vi "Karma License Activator.vi"() -> ()   [LabVIEW 2022 SP3]
panel:
  in  "Activate License":bool
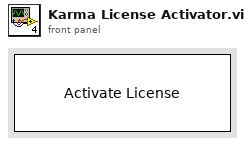
[diagram p1: front panel]
types:
  T1 = enum16{"open", "replace", "create", "open or create", "replace or create", "replace or create with confirmation"}
  T2 = typedef "Paths.ctl" = cluster{"Configuration":path, "Event Logs":path, "Error Logs":path, "Configuration.ini":path}
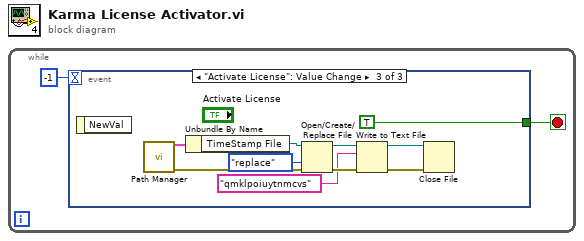
[diagram p0: block diagram]
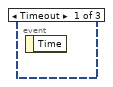
[diagram p2: hidden frame]
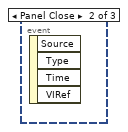
[diagram p3: hidden frame]
diagram:
  n1 = while {
    stop <- w1 stop-if-true
    n2 = event shown="[2] \"Activate License\": Value Change" {
      selector: _ -> [_ _ _]
      dyn-events: _ -> [_ _ _]
      timeout: -1 -> [_ _ _]
      tunnel: [_ _ TRUE] -> w1
      event Timeout {
        n3 = event-data() -> ()  [unwired: 1 in, 1 out]
      }
      event Panel Close {
        n4 = event-data() -> ()  [unwired: 1 in, 4 out]
      }
      event "Activate License": Value Change {
        n5 = event-data() -> ()  [unwired: 1 in, 1 out]
        n6 = call "Path Manager.vi"() -> ("Cluster"=w10:T2, "Error out"=w9:errorcluster)  [unwired: 14 in]
        n7 = Unbundle By Name(w10) -> ("TimeStamp File"=w8:path)
        n8 = Open/Create/Replace File(file path (use dialog)=w8, error in=w9, operation (0:open)=T1."replace") -> (refnum out=w6:refnum<file>, error out=w11:errorcluster)  [unwired: 3 in, 1 out]
        n9 = Write to Text File(file (use dialog)=w6, text="qmklpoiuytnmcvs") -> (refnum out=w5:refnum<file>)  [unwired: 2 in, 2 out]
        n10 = Close File(refnum=w5, error in=w11) -> ()  [unwired: 2 out]
      }
    }
  }
